vi "_시리얼_Mark10-제어 (압력설정).vi"(3 "FTS 제어 상태":T1="압력제어 시작", 4 "압력 설정(lb)":dbl=10.0 min=0.0 max=160.0 step=0.01 format="%.2f", 5 "시리얼 포트":refnum<visa-resource-name>="COM5") -> (0 "게이지 압력(lb)":dbl min=0.0 max=160.0 step=0.01 format="%.2f", 1 "통신 정상":bool=TRUE, 2 "시리얼 포트out":refnum<visa-resource-name>="COM5")   [LabVIEW 2015]
panel:
  out "미세조정 횟수":u32
  in  "속도-미세조정(mm/min)":dbl=1.0
  in  "속도-저속(mm/min)":dbl=4.0
  in  "속도-중속(mm/min)":dbl=60.0
  in  "속도-고속(mm/min)":dbl=250.0
  # "MARK10 압력 제어"
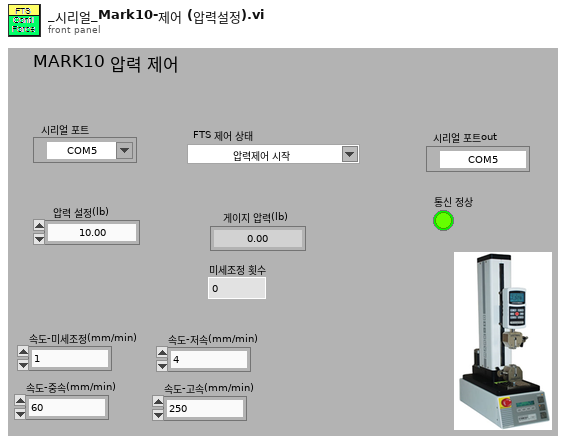
[diagram p1: front panel]
types:
  T1 = typedef "컨트롤-동작상태 FTS.ctl" = string
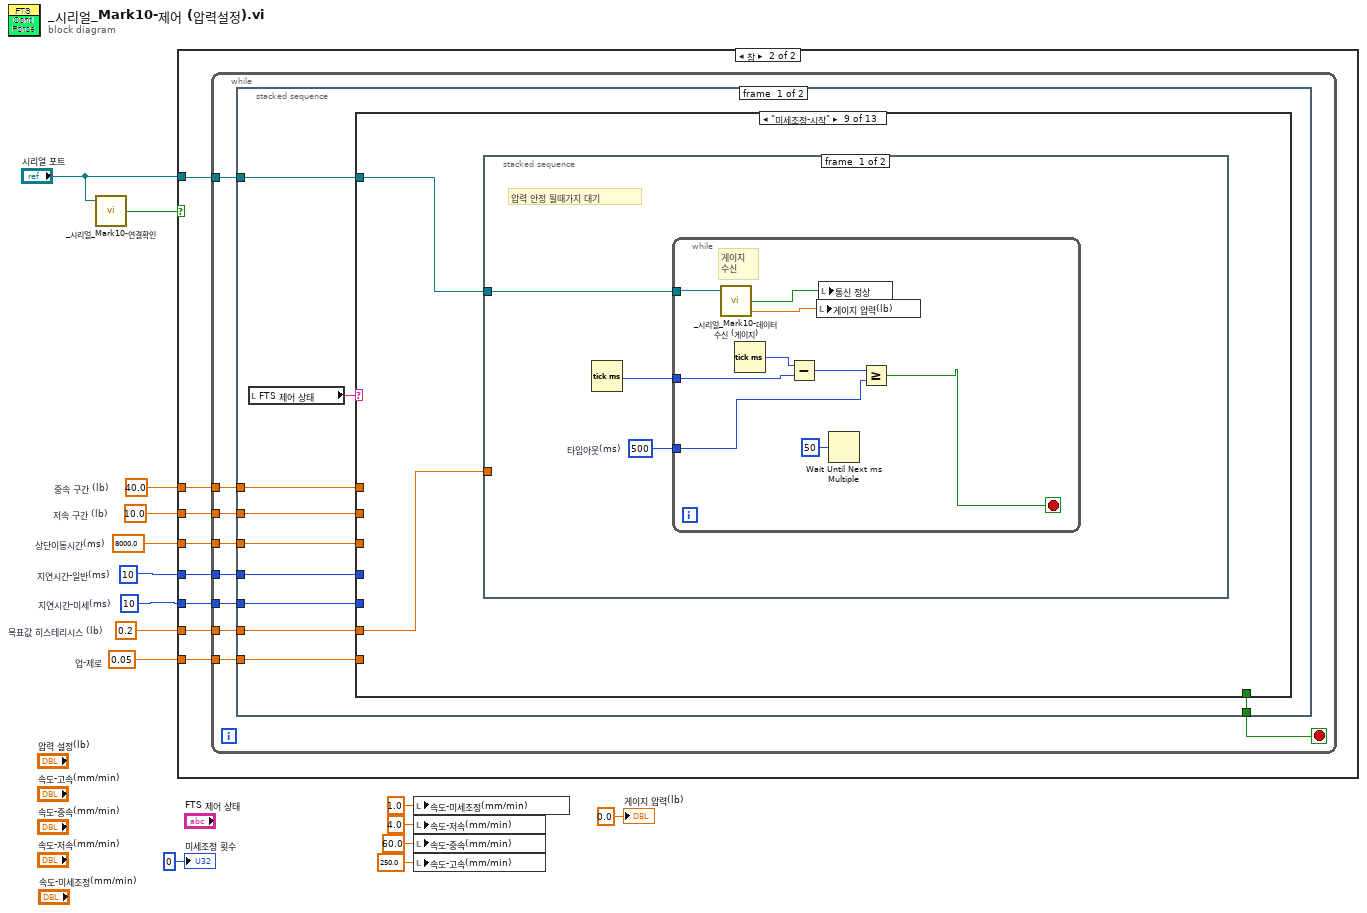
[diagram p0: block diagram]
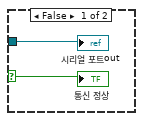
[diagram p2: hidden frame]
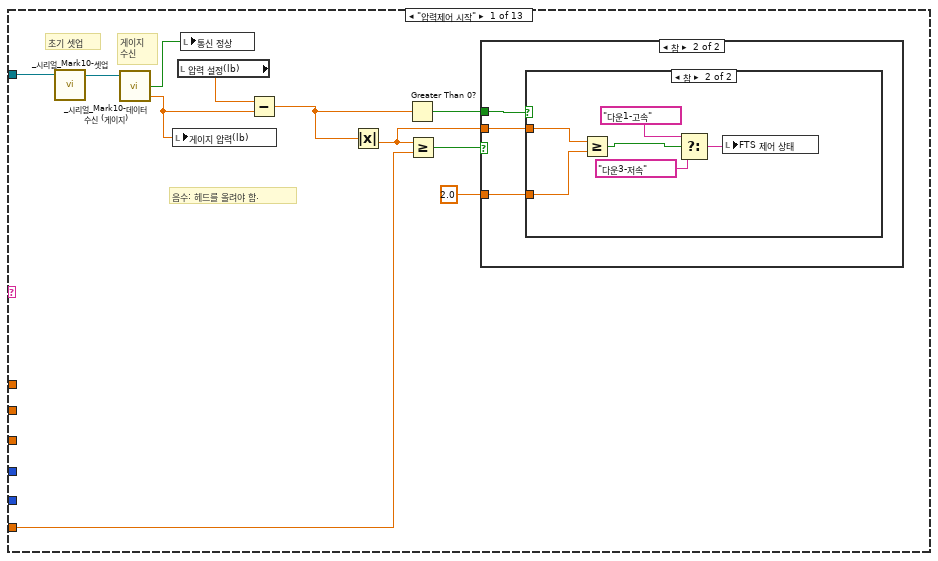
[diagram p3: hidden frame]
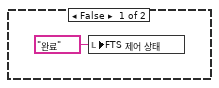
[diagram p4: hidden frame]
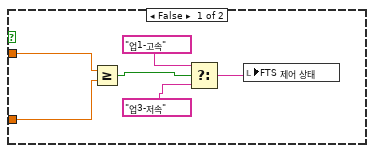
[diagram p5: hidden frame]
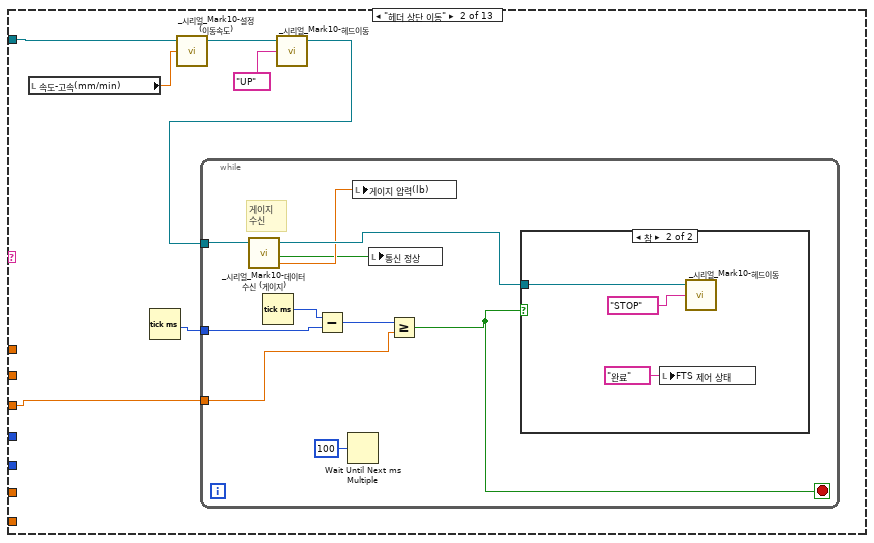
[diagram p6: hidden frame]
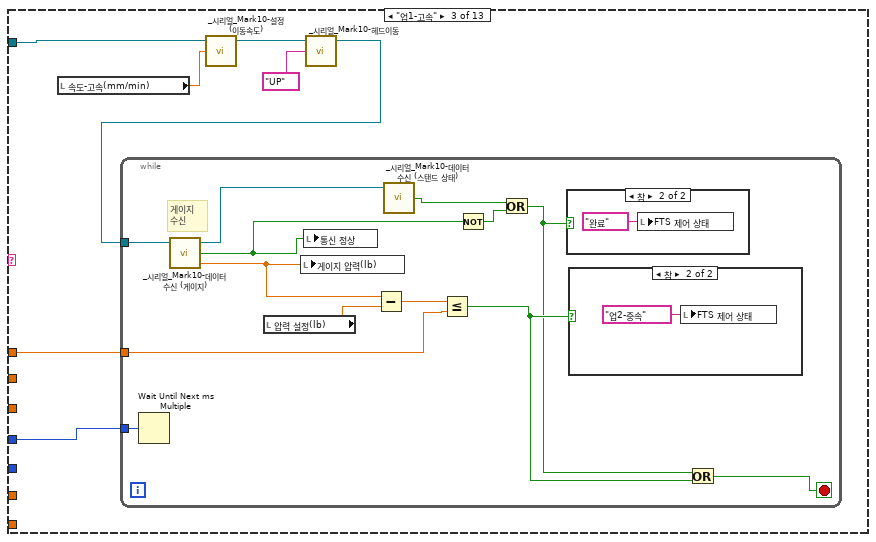
[diagram p8: hidden frame]
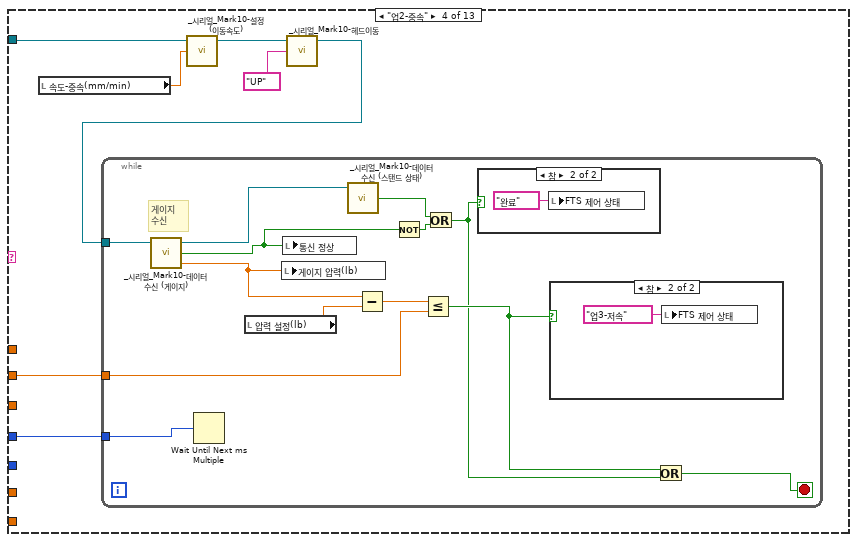
[diagram p11: hidden frame]
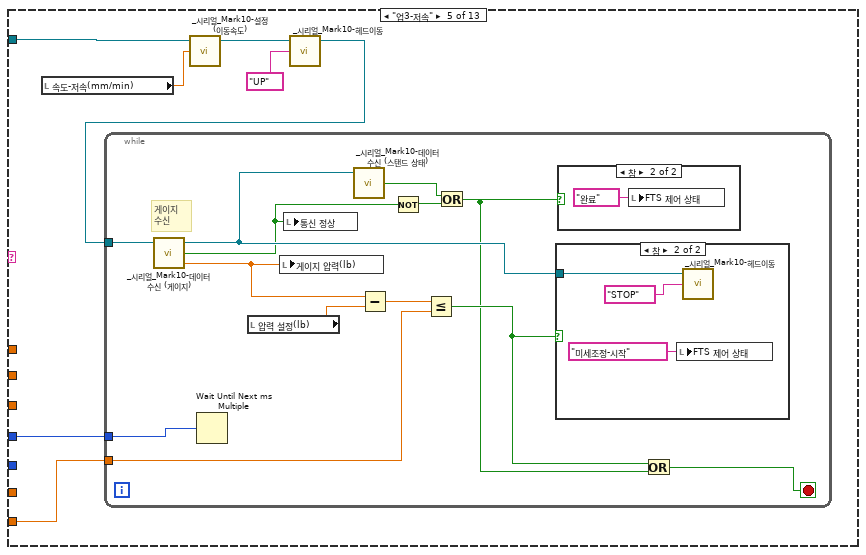
[diagram p14: hidden frame]
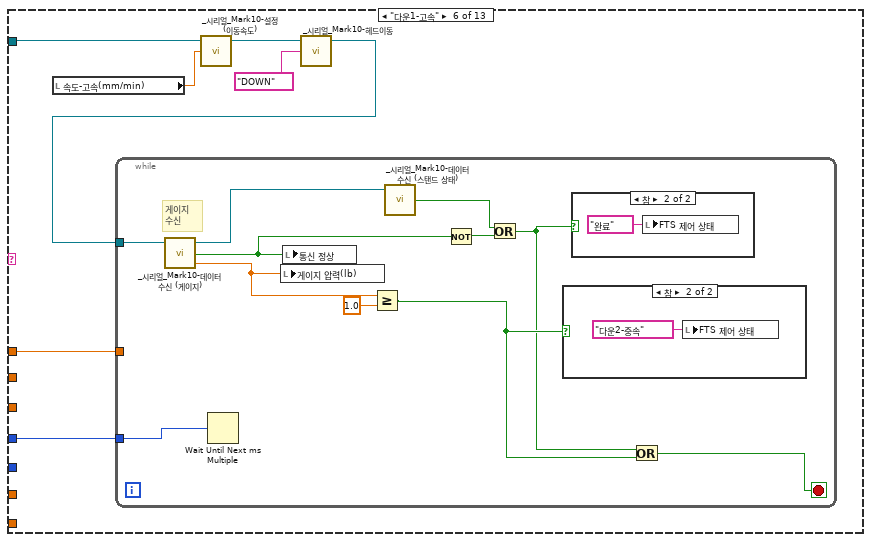
[diagram p17: hidden frame]
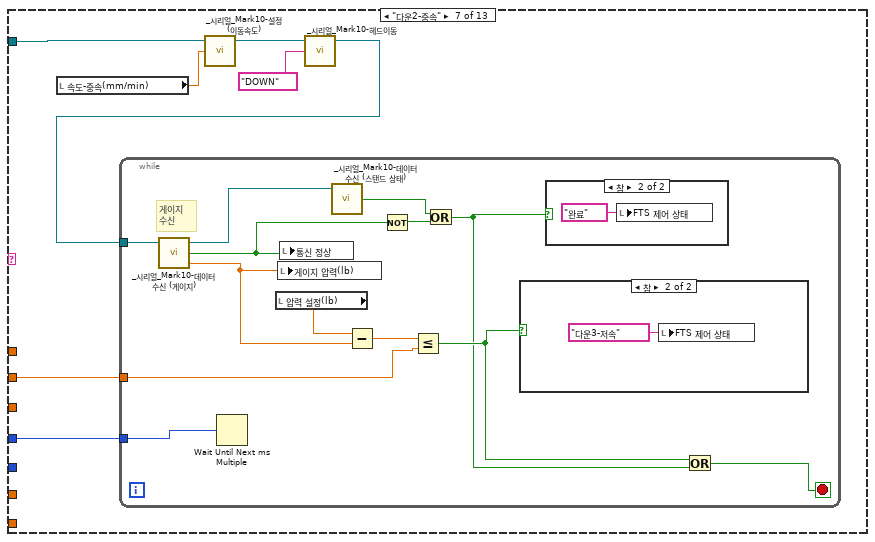
[diagram p20: hidden frame]
diagram:
  w1 = 0.05  # 업-제로
  w3 = 0.2  # 목표값 히스테리시스 (lb)
  w8 = u32 10  # 지연시간-미세(ms)
  w9 = u32 10  # 지연시간-일반(ms)
  w10 = 8000.0  # 상단이동시간(ms)
  w11 = 10.0  # 저속 구간 (lb)
  w12 = 40.0  # 중속 구간 (lb)
  n1 = call "_시리얼_Mark10-연결확인.vi"("시리얼 포트"="시리얼 포트") -> ("수신 정상"=w13:bool)  [unwired: 3 in, 1 out]
  n2 = case shown="참" w13 {
    selector: w13 -> [w16 _]
    tunnel: "시리얼 포트" -> [w17 w25]
    tunnel: w12 -> [_ w24]
    tunnel: w11 -> [_ w23]
    tunnel: w10 -> [_ w22]
    tunnel: w9 -> [_ w21]
    tunnel: w8 -> [_ w20]
    tunnel: w3 -> [_ w19]
    tunnel: w1 -> [_ w18]
    frame False {
      "통신 정상" <- w16
      "시리얼 포트out" <- w17
    }
    frame True {
      n3 = while {
        tunnel: w25 -> [w34]
        tunnel: w24 -> [w32]
        tunnel: w23 -> [w31]
        tunnel: w22 -> [w30]
        tunnel: w21 -> [w29]
        tunnel: w20 -> [w28]
        tunnel: w19 -> [w27]
        tunnel: w18 -> [w26]
        stop <- w33 stop-if-true
        n4 = stacked-sequence {
          tunnel: w34 -> [w44 _]
          tunnel: [w42 _] -> w33
          tunnel: w32 -> [w41 _]
          tunnel: w31 -> [w40 _]
          tunnel: w30 -> [w39 _]
          tunnel: w29 -> [w38 _]
          tunnel: w28 -> [w37 _]
          tunnel: w27 -> [w36 _]
          tunnel: w26 -> [w35 _]
          frame #0 {
            n5 = local read "FTS 제어 상태"() -> (w43:T1)
            n6 = case shown="\"미세조정-시작\"" w43 {
              tunnel: w44 -> [w55 w74 w94 w116 w138 w165 w182 w203 w226 w254 w279 w304 w325]
              tunnel: [_ _ _ _ _ _ _ _ _ _ _ _ TRUE] -> w42
              tunnel: w41 -> [_ _ w93 _ _ w161 _ _ _ _ _ _ _]
              tunnel: w40 -> [_ _ _ w115 _ _ w181 _ _ _ _ _ _]
              tunnel: w39 -> [_ w72 _ _ _ _ _ _ _ _ _ _ _]
              tunnel: w38 -> [_ _ w92 w114 w137 w160 w180 w202 _ _ _ _ _]
              tunnel: w37 -> [_ _ _ _ _ _ _ _ _ w253 w278 _ _]
              tunnel: w36 -> [w45 _ _ _ _ _ _ _ w225 _ _ w303 _]
              tunnel: w35 -> [_ _ _ _ w136 _ _ _ _ _ w277 _ _]
              frame "압력제어 시작" {
                # "음수: 헤드를 올려야 함."
                # "게이지\n수신"
                # "초기 셋업"
                n7 = call "_시리얼_Mark10-셋업.vi"("시리얼 포트"=w55) -> ("VISA 리소스 이름 출력"=w54:refnum<visa-resource-name>)  [unwired: 4 in]
                n8 = call "_시리얼_Mark10-데이터 수신 (게이지).vi"("시리얼 포트"=w54) -> ("데이터(lb)"=w52:dbl, "수신 정상"=w46:bool)  [unwired: 2 in, 1 out]
                n9 = local write "게이지 압력(lb)"(w52) -> ()
                n10 = local read "압력 설정(lb)"() -> (w53:dbl)
                n11 = local write "통신 정상"(w46) -> ()
                n12 = Subtract(x=w53, y=w52) -> (x-y=w50:dbl)
                n13 = Absolute Value(x=w50) -> (abs(x)=w48:dbl)
                n14 = Greater Than 0?(x=w50) -> (x > 0?=w49:bool)
                n15 = Greater Or Equal?(x=w48, y=w45) -> (x >= y?=w51:bool)
                n16 = case shown="참" w51 {
                  tunnel: w49 -> [_ w59]
                  tunnel: w48 -> [_ w58]
                  tunnel: 2.0 ("y") -> [_ w57]
                  frame False {
                    n17 = local write "FTS 제어 상태"(T1 "완료" ("FTS 제어 상태")) -> ()
                  }
                  frame True {
                    n18 = case shown="참" w59 {
                      tunnel: w58 -> [w62 w71]
                      tunnel: w57 -> [w60 w67]
                      frame False {
                        n19 = Greater Or Equal?(x=w62, y=w60) -> (x >= y?=w65:bool)
                        n20 = Select(t=T1 "업1-고속" ("FTS 제어 상태"), s=w65, f=T1 "업3-저속" ("FTS 제어 상태")) -> (s? t:f=w61:T1)
                        n21 = local write "FTS 제어 상태"(w61) -> ()
                      }
                      frame True {
                        n22 = Greater Or Equal?(x=w71, y=w67) -> (x >= y?=w70:bool)
                        n23 = Select(t=T1 "다운1-고속" ("FTS 제어 상태"), s=w70, f=T1 "다운3-저속") -> (s? t:f=w68:T1)
                        n24 = local write "FTS 제어 상태"(w68) -> ()
                      }
                    }
                  }
                }
              }
              frame "헤더 상단 이동" {
                n25 = local read "속도-고속(mm/min)"() -> (w78:dbl)
                n26 = Tick Count (ms)() -> (millisecond timer value=w73:u32)
                n27 = call "_시리얼_Mark10-설정 (이동속도).vi"("속도(mm/min)"=w78, "시리얼 포트"=w74) -> ("VISA 리소스 이름 출력"=w76:refnum<visa-resource-name>)  [unwired: 3 in]
                n28 = call "_시리얼_Mark10-헤드이동.vi"("동작 모드"="UP", "시리얼 포트"=w76) -> ("VISA 리소스 이름 출력"=w75:refnum<visa-resource-name>)  [unwired: 3 in]
                n29 = while {
                  tunnel: w75 -> [w88]
                  tunnel: w73 -> [w83]
                  tunnel: w72 -> [w81]
                  stop <- w80 stop-if-true
                  # "게이지\n수신"
                  n30 = call "_시리얼_Mark10-데이터 수신 (게이지).vi"("시리얼 포트"=w88) -> ("데이터(lb)"=w85:dbl, "수신 정상"=w79:bool, "시리얼 포트 out"=w87:refnum<visa-resource-name>)  [unwired: 2 in]
                  n31 = Tick Count (ms)() -> (millisecond timer value=w84:u32)
                  n32 = Subtract(x=w84, y=w83) -> (x-y=w82:u32)
                  n33 = Wait Until Next ms Multiple(millisecond multiple=u32 100 ("ms 배수")) -> ()  [unwired: 1 out]
                  n34 = local write "게이지 압력(lb)"(w85) -> ()
                  n35 = local write "통신 정상"(w79) -> ()
                  n36 = Greater Or Equal?(x=w82, y=w81) -> (x >= y?=w80:bool)
                  n37 = case shown="참" w80 {
                    tunnel: w87 -> [_ w89]
                    frame False {
                    }
                    frame True {
                      n38 = local write "FTS 제어 상태"(T1 "완료" ("FTS 제어 상태")) -> ()
                      n39 = call "_시리얼_Mark10-헤드이동.vi"("동작 모드"="STOP", "시리얼 포트"=w89) -> ()  [unwired: 3 in, 1 out]
                    }
                  }
                }
              }
              frame "업1-고속" {
                n40 = local read "속도-고속(mm/min)"() -> (w98:dbl)
                n41 = call "_시리얼_Mark10-설정 (이동속도).vi"("속도(mm/min)"=w98, "시리얼 포트"=w94) -> ("VISA 리소스 이름 출력"=w96:refnum<visa-resource-name>)  [unwired: 3 in]
                n42 = call "_시리얼_Mark10-헤드이동.vi"("동작 모드"="UP", "시리얼 포트"=w96) -> ("VISA 리소스 이름 출력"=w95:refnum<visa-resource-name>)  [unwired: 3 in]
                n43 = while {
                  tunnel: w95 -> [w111]
                  tunnel: w93 -> [w107]
                  tunnel: w92 -> [w106]
                  stop <- w103 stop-if-true
                  # "게이지\n수신"
                  n44 = Wait Until Next ms Multiple(millisecond multiple=w106) -> ()  [unwired: 1 out]
                  n45 = call "_시리얼_Mark10-데이터 수신 (게이지).vi"("시리얼 포트"=w111) -> ("데이터(lb)"=w108:dbl, "수신 정상"=w99:bool, "시리얼 포트 out"=w105:refnum<visa-resource-name>)  [unwired: 2 in]
                  n46 = local read "압력 설정(lb)"() -> (w110:dbl)
                  n47 = local write "게이지 압력(lb)"(w108) -> ()
                  n48 = local write "통신 정상"(w99) -> ()
                  n49 = Subtract(x=w108, y=w110) -> (x-y=w109:dbl)
                  n50 = call "_시리얼_Mark10-데이터 수신 (스탠드 상태).vi"("시리얼 포트"=w105) -> ("모터 정지 상태"=w101:bool)  [unwired: 3 in, 1 out]
                  n51 = Less Or Equal?(x=w109, y=w107) -> (x <= y?=w104:bool)
                  n52 = Not(x=w99) -> (.not. x?=w100:bool)
                  n53 = Or(x=w101, y=w100) -> (x .or. y?=w102:bool)
                  n54 = case shown="참" w102 {
                    frame False {
                    }
                    frame True {
                      n55 = local write "FTS 제어 상태"(T1 "완료" ("FTS 제어 상태")) -> ()
                    }
                  }
                  n56 = case shown="참" w104 {
                    frame False {
                    }
                    frame True {
                      n57 = local write "FTS 제어 상태"(T1 "업2-중속" ("FTS 제어 상태")) -> ()
                    }
                  }
                  n58 = Or(x=w102, y=w104) -> (x .or. y?=w103:bool)
                }
              }
              frame "업2-중속" {
                n59 = local read "속도-중속(mm/min)"() -> (w120:dbl)
                n60 = call "_시리얼_Mark10-설정 (이동속도).vi"("속도(mm/min)"=w120, "시리얼 포트"=w116) -> ("VISA 리소스 이름 출력"=w118:refnum<visa-resource-name>)  [unwired: 3 in]
                n61 = call "_시리얼_Mark10-헤드이동.vi"("동작 모드"="UP", "시리얼 포트"=w118) -> ("VISA 리소스 이름 출력"=w117:refnum<visa-resource-name>)  [unwired: 3 in]
                n62 = while {
                  tunnel: w117 -> [w133]
                  tunnel: w115 -> [w129]
                  tunnel: w114 -> [w128]
                  stop <- w125 stop-if-true
                  # "게이지\n수신"
                  n63 = call "_시리얼_Mark10-데이터 수신 (게이지).vi"("시리얼 포트"=w133) -> ("데이터(lb)"=w130:dbl, "수신 정상"=w121:bool, "시리얼 포트 out"=w127:refnum<visa-resource-name>)  [unwired: 2 in]
                  n64 = Wait Until Next ms Multiple(millisecond multiple=w128) -> ()  [unwired: 1 out]
                  n65 = local read "압력 설정(lb)"() -> (w132:dbl)
                  n66 = local write "게이지 압력(lb)"(w130) -> ()
                  n67 = local write "통신 정상"(w121) -> ()
                  n68 = call "_시리얼_Mark10-데이터 수신 (스탠드 상태).vi"("시리얼 포트"=w127) -> ("모터 정지 상태"=w123:bool)  [unwired: 3 in, 1 out]
                  n69 = Subtract(x=w130, y=w132) -> (x-y=w131:dbl)
                  n70 = Not(x=w121) -> (.not. x?=w124:bool)
                  n71 = Less Or Equal?(x=w131, y=w129) -> (x <= y?=w126:bool)
                  n72 = Or(x=w123, y=w124) -> (x .or. y?=w122:bool)
                  n73 = case shown="참" w122 {
                    frame False {
                    }
                    frame True {
                      n74 = local write "FTS 제어 상태"(T1 "완료" ("FTS 제어 상태")) -> ()
                    }
                  }
                  n75 = case shown="참" w126 {
                    frame False {
                    }
                    frame True {
                      n76 = local write "FTS 제어 상태"(T1 "업3-저속" ("FTS 제어 상태")) -> ()
                    }
                  }
                  n77 = Or(x=w126, y=w122) -> (x .or. y?=w125:bool)
                }
              }
              frame "업3-저속" {
                n78 = local read "속도-저속(mm/min)"() -> (w142:dbl)
                n79 = call "_시리얼_Mark10-설정 (이동속도).vi"("속도(mm/min)"=w142, "시리얼 포트"=w138) -> ("VISA 리소스 이름 출력"=w140:refnum<visa-resource-name>)  [unwired: 3 in]
                n80 = call "_시리얼_Mark10-헤드이동.vi"("동작 모드"="UP", "시리얼 포트"=w140) -> ("VISA 리소스 이름 출력"=w139:refnum<visa-resource-name>)  [unwired: 3 in]
                n81 = while {
                  tunnel: w139 -> [w155]
                  tunnel: w137 -> [w151]
                  tunnel: w136 -> [w143]
                  stop <- w148 stop-if-true
                  # "게이지\n수신"
                  n82 = call "_시리얼_Mark10-데이터 수신 (게이지).vi"("시리얼 포트"=w155) -> ("데이터(lb)"=w152:dbl, "수신 정상"=w147:bool, "시리얼 포트 out"=w150:refnum<visa-resource-name>)  [unwired: 2 in]
                  n83 = Wait Until Next ms Multiple(millisecond multiple=w151) -> ()  [unwired: 1 out]
                  n84 = local read "압력 설정(lb)"() -> (w154:dbl)
                  n85 = local write "게이지 압력(lb)"(w152) -> ()
                  n86 = local write "통신 정상"(w147) -> ()
                  n87 = call "_시리얼_Mark10-데이터 수신 (스탠드 상태).vi"("시리얼 포트"=w150) -> ("모터 정지 상태"=w145:bool)  [unwired: 3 in, 1 out]
                  n88 = Subtract(x=w152, y=w154) -> (x-y=w153:dbl)
                  n89 = Not(x=w147) -> (.not. x?=w146:bool)
                  n90 = Less Or Equal?(x=w153, y=w143) -> (x <= y?=w149:bool)
                  n91 = Or(x=w145, y=w146) -> (x .or. y?=w144:bool)
                  n92 = case shown="참" w149 {
                    tunnel: w150 -> [_ w158]
                    frame False {
                    }
                    frame True {
                      n93 = local write "FTS 제어 상태"(T1 "미세조정-시작" ("FTS 제어 상태")) -> ()
                      n94 = call "_시리얼_Mark10-헤드이동.vi"("동작 모드"="STOP", "시리얼 포트"=w158) -> ()  [unwired: 3 in, 1 out]
                    }
                  }
                  n95 = case shown="참" w144 {
                    frame False {
                    }
                    frame True {
                      n96 = local write "FTS 제어 상태"(T1 "완료" ("FTS 제어 상태")) -> ()
                    }
                  }
                  n97 = Or(x=w149, y=w144) -> (x .or. y?=w148:bool)
                }
              }
              frame "다운1-고속" {
                n98 = local read "속도-고속(mm/min)"() -> (w166:dbl)
                n99 = call "_시리얼_Mark10-설정 (이동속도).vi"("속도(mm/min)"=w166, "시리얼 포트"=w165) -> ("VISA 리소스 이름 출력"=w163:refnum<visa-resource-name>)  [unwired: 3 in]
                n100 = call "_시리얼_Mark10-헤드이동.vi"("동작 모드"="DOWN", "시리얼 포트"=w163) -> ("VISA 리소스 이름 출력"=w162:refnum<visa-resource-name>)  [unwired: 3 in]
                n101 = while {
                  tunnel: w162 -> [w177]
                  tunnel: w161 -> [_]
                  tunnel: w160 -> [w174]
                  stop <- w171 stop-if-true
                  # "게이지\n수신"
                  n102 = call "_시리얼_Mark10-데이터 수신 (게이지).vi"("시리얼 포트"=w177) -> ("데이터(lb)"=w176:dbl, "수신 정상"=w170:bool, "시리얼 포트 out"=w173:refnum<visa-resource-name>)  [unwired: 2 in]
                  n103 = Wait Until Next ms Multiple(millisecond multiple=w174) -> ()  [unwired: 1 out]
                  n104 = local write "게이지 압력(lb)"(w176) -> ()
                  n105 = local write "통신 정상"(w170) -> ()
                  n106 = Greater Or Equal?(x=w176, y=1.0) -> (x >= y?=w172:bool)
                  n107 = call "_시리얼_Mark10-데이터 수신 (스탠드 상태).vi"("시리얼 포트"=w173) -> ("모터 정지 상태"=w168:bool)  [unwired: 3 in, 1 out]
                  n108 = Not(x=w170) -> (.not. x?=w169:bool)
                  n109 = Or(x=w168, y=w169) -> (x .or. y?=w167:bool)
                  n110 = case shown="참" w172 {
                    frame False {
                    }
                    frame True {
                      n111 = local write "FTS 제어 상태"(T1 "다운2-중속" ("FTS 제어 상태")) -> ()
                    }
                  }
                  n112 = case shown="참" w167 {
                    frame False {
                    }
                    frame True {
                      n113 = local write "FTS 제어 상태"(T1 "완료" ("FTS 제어 상태")) -> ()
                    }
                  }
                  n114 = Or(x=w167, y=w172) -> (x .or. y?=w171:bool)
                }
              }
              frame "다운2-중속" {
                n115 = local read "속도-중속(mm/min)"() -> (w186:dbl)
                n116 = call "_시리얼_Mark10-설정 (이동속도).vi"("속도(mm/min)"=w186, "시리얼 포트"=w182) -> ("VISA 리소스 이름 출력"=w184:refnum<visa-resource-name>)  [unwired: 3 in]
                n117 = call "_시리얼_Mark10-헤드이동.vi"("동작 모드"="DOWN", "시리얼 포트"=w184) -> ("VISA 리소스 이름 출력"=w183:refnum<visa-resource-name>)  [unwired: 3 in]
                n118 = while {
                  tunnel: w183 -> [w199]
                  tunnel: w181 -> [w195]
                  tunnel: w180 -> [w194]
                  stop <- w191 stop-if-true
                  # "게이지\n수신"
                  n119 = call "_시리얼_Mark10-데이터 수신 (게이지).vi"("시리얼 포트"=w199) -> ("데이터(lb)"=w196:dbl, "수신 정상"=w190:bool, "시리얼 포트 out"=w193:refnum<visa-resource-name>)  [unwired: 2 in]
                  n120 = Wait Until Next ms Multiple(millisecond multiple=w194) -> ()  [unwired: 1 out]
                  n121 = local read "압력 설정(lb)"() -> (w198:dbl)
                  n122 = local write "게이지 압력(lb)"(w196) -> ()
                  n123 = local write "통신 정상"(w190) -> ()
                  n124 = call "_시리얼_Mark10-데이터 수신 (스탠드 상태).vi"("시리얼 포트"=w193) -> ("모터 정지 상태"=w188:bool)  [unwired: 3 in, 1 out]
                  n125 = Subtract(x=w198, y=w196) -> (x-y=w197:dbl)
                  n126 = Not(x=w190) -> (.not. x?=w189:bool)
                  n127 = Less Or Equal?(x=w197, y=w195) -> (x <= y?=w192:bool)
                  n128 = Or(x=w188, y=w189) -> (x .or. y?=w187:bool)
                  n129 = case shown="참" w192 {
                    frame False {
                    }
                    frame True {
                      n130 = local write "FTS 제어 상태"(T1 "다운3-저속" ("FTS 제어 상태")) -> ()
                    }
                  }
                  n131 = case shown="참" w187 {
                    frame False {
                    }
                    frame True {
                      n132 = local write "FTS 제어 상태"(T1 "완료" ("FTS 제어 상태")) -> ()
                    }
                  }
                  n133 = Or(x=w192, y=w187) -> (x .or. y?=w191:bool)
                }
              }
              frame "다운3-저속" {
                n134 = local read "속도-저속(mm/min)"() -> (w207:dbl)
                n135 = call "_시리얼_Mark10-설정 (이동속도).vi"("속도(mm/min)"=w207, "시리얼 포트"=w203) -> ("VISA 리소스 이름 출력"=w205:refnum<visa-resource-name>)  [unwired: 3 in]
                n136 = call "_시리얼_Mark10-헤드이동.vi"("동작 모드"="DOWN", "시리얼 포트"=w205) -> ("VISA 리소스 이름 출력"=w204:refnum<visa-resource-name>)  [unwired: 3 in]
                n137 = while {
                  tunnel: w204 -> [w220]
                  tunnel: w202 -> [w216]
                  stop <- w214 stop-if-true
                  # "게이지\n수신"
                  n138 = call "_시리얼_Mark10-데이터 수신 (게이지).vi"("시리얼 포트"=w220) -> ("데이터(lb)"=w217:dbl, "수신 정상"=w208:bool, "시리얼 포트 out"=w213:refnum<visa-resource-name>)  [unwired: 2 in]
                  n139 = Wait Until Next ms Multiple(millisecond multiple=w216) -> ()  [unwired: 1 out]
                  n140 = local write "통신 정상"(w208) -> ()
                  n141 = local read "압력 설정(lb)"() -> (w219:dbl)
                  n142 = local write "게이지 압력(lb)"(w217) -> ()
                  n143 = Subtract(x=w219, y=w217) -> (x-y=w218:dbl)
                  n144 = call "_시리얼_Mark10-데이터 수신 (스탠드 상태).vi"("시리얼 포트"=w213) -> ("모터 정지 상태"=w211:bool, "시리얼 포트 out"=w212:refnum<visa-resource-name>)  [unwired: 3 in]
                  n145 = Less Or Equal To 0?(x=w218) -> (x <= 0?=w215:bool)
                  n146 = Not(x=w208) -> (.not. x?=w210:bool)
                  n147 = Or(x=w211, y=w210) -> (x .or. y?=w209:bool)
                  n148 = case shown="참" w215 {
                    tunnel: w212 -> [_ w223]
                    frame False {
                    }
                    frame True {
                      n149 = local write "FTS 제어 상태"(T1 "미세조정-시작" ("FTS 제어 상태")) -> ()
                      n150 = call "_시리얼_Mark10-헤드이동.vi"("동작 모드"="STOP", "시리얼 포트"=w223) -> ()  [unwired: 3 in, 1 out]
                    }
                  }
                  n151 = case shown="참" w209 {
                    frame False {
                    }
                    frame True {
                      n152 = local write "FTS 제어 상태"(T1 "완료" ("FTS 제어 상태")) -> ()
                    }
                  }
                  n153 = Or(x=w215, y=w209) -> (x .or. y?=w214:bool)
                }
              }
              frame "미세조정-시작" {
                n154 = stacked-sequence {
                  tunnel: w226 -> [w229 w247]
                  tunnel: w225 -> [_ w244]
                  frame #0 {
                    w227 = u32 500  # 타임아웃(ms)
                    # "압력 안정 될때가지 대기"
                    n155 = Tick Count (ms)() -> (millisecond timer value=w228:u32)
                    n156 = while {
                      tunnel: w229 -> [w238]
                      tunnel: w228 -> [w234]
                      tunnel: w227 -> [w232]
                      stop <- w231 stop-if-true
                      # "게이지\n수신"
                      n157 = call "_시리얼_Mark10-데이터 수신 (게이지).vi"("시리얼 포트"=w238) -> ("데이터(lb)"=w236:dbl, "수신 정상"=w230:bool)  [unwired: 2 in, 1 out]
                      n158 = Tick Count (ms)() -> (millisecond timer value=w235:u32)
                      n159 = Subtract(x=w235, y=w234) -> (x-y=w233:u32)
                      n160 = local write "게이지 압력(lb)"(w236) -> ()
                      n161 = local write "통신 정상"(w230) -> ()
                      n162 = Wait Until Next ms Multiple(millisecond multiple=u32 50 ("ms 배수")) -> ()  [unwired: 1 out]
                      n163 = Greater Or Equal?(x=w233, y=w232) -> (x >= y?=w231:bool)
                    }
                  }
                  frame #1 {
                    # "음수: 헤드를 올려야 함."
                    # "게이지\n수신"
                    n164 = call "_시리얼_Mark10-데이터 수신 (게이지).vi"("시리얼 포트"=w247) -> ("데이터(lb)"=w248:dbl, "수신 정상"=w246:bool)  [unwired: 2 in, 1 out]
                    n165 = local write "게이지 압력(lb)"(w248) -> ()
                    n166 = local read "압력 설정(lb)"() -> (w249:dbl)
                    n167 = local write "통신 정상"(w246) -> ()
                    n168 = Subtract(x=w249, y=w248) -> (x-y=w245:dbl)
                    n169 = Multiply(x=w244, y=-1.0) -> (x*y=w243:dbl)
                    n170 = Greater Or Equal?(x=w245, y=w244) -> (x >= y?=w240:bool)
                    n171 = Less Or Equal?(x=w245, y=w243) -> (x <= y?=w241:bool)
                    n172 = Or(x=w241, y=w240) -> (x .or. y?=w239:bool)
                    n173 = case shown="참" w240 {
                      frame False {
                      }
                      frame True {
                        n174 = local write "FTS 제어 상태"(T1 "미세조정-다운" ("FTS 제어 상태")) -> ()
                      }
                    }
                    n175 = case shown="참" w241 {
                      frame False {
                      }
                      frame True {
                        n176 = local write "FTS 제어 상태"(T1 "미세조정-업" ("FTS 제어 상태")) -> ()
                      }
                    }
                    n177 = case shown="거짓" w239 {
                      frame False {
                        n178 = local write "FTS 제어 상태"(T1 "미세조정-종료" ("FTS 제어 상태")) -> ()
                      }
                      frame True {
                      }
                    }
                  }
                }
              }
              frame "미세조정-다운" {
                n179 = local read "속도-미세조정(mm/min)"() -> (w258:dbl)
                n180 = call "_시리얼_Mark10-설정 (이동속도).vi"("속도(mm/min)"=w258, "시리얼 포트"=w254) -> ("VISA 리소스 이름 출력"=w256:refnum<visa-resource-name>)  [unwired: 3 in]
                n181 = call "_시리얼_Mark10-헤드이동.vi"("동작 모드"="DOWN", "시리얼 포트"=w256) -> ("VISA 리소스 이름 출력"=w255:refnum<visa-resource-name>)  [unwired: 3 in]
                n182 = while {
                  tunnel: w255 -> [w271]
                  tunnel: w253 -> [w265]
                  stop <- w266 stop-if-true
                  # "게이지\n수신"
                  n183 = call "_시리얼_Mark10-데이터 수신 (게이지).vi"("시리얼 포트"=w271) -> ("데이터(lb)"=w268:dbl, "수신 정상"=w259:bool, "시리얼 포트 out"=w264:refnum<visa-resource-name>)  [unwired: 2 in]
                  n184 = local write "통신 정상"(w259) -> ()
                  n185 = local read "압력 설정(lb)"() -> (w270:dbl)
                  n186 = local write "게이지 압력(lb)"(w268) -> ()
                  n187 = call "_시리얼_Mark10-데이터 수신 (스탠드 상태).vi"("시리얼 포트"=w264) -> ("모터 정지 상태"=w261:bool, "시리얼 포트 out"=w263:refnum<visa-resource-name>)  [unwired: 3 in]
                  n188 = Subtract(x=w270, y=w268) -> (x-y=w269:dbl)
                  n189 = Not(x=w259) -> (.not. x?=w262:bool)
                  n190 = Less Or Equal To 0?(x=w269) -> (x <= 0?=w267:bool)
                  n191 = Or(x=w261, y=w262) -> (x .or. y?=w260:bool)
                  n192 = case shown="참" w267 {
                    tunnel: w263 -> [_ w275]
                    tunnel: w265 -> [w273 _]
                    frame False {
                      n193 = Wait Until Next ms Multiple(millisecond multiple=w273) -> ()  [unwired: 1 out]
                    }
                    frame True {
                      n194 = local write "FTS 제어 상태"(T1 "미세조정-종료" ("FTS 제어 상태")) -> ()
                      n195 = call "_시리얼_Mark10-헤드이동.vi"("동작 모드"="STOP", "시리얼 포트"=w275) -> ()  [unwired: 3 in, 1 out]
                    }
                  }
                  n196 = case shown="참" w260 {
                    frame False {
                    }
                    frame True {
                      n197 = local write "FTS 제어 상태"(T1 "완료" ("FTS 제어 상태")) -> ()
                    }
                  }
                  n198 = Or(x=w267, y=w260) -> (x .or. y?=w266:bool)
                }
              }
              frame "미세조정-업" {
                n199 = local read "속도-저속(mm/min)"() -> (w283:dbl)
                n200 = call "_시리얼_Mark10-설정 (이동속도).vi"("속도(mm/min)"=w283, "시리얼 포트"=w279) -> ("VISA 리소스 이름 출력"=w281:refnum<visa-resource-name>)  [unwired: 3 in]
                n201 = call "_시리얼_Mark10-헤드이동.vi"("동작 모드"="UP", "시리얼 포트"=w281) -> ("VISA 리소스 이름 출력"=w280:refnum<visa-resource-name>)  [unwired: 3 in]
                n202 = while {
                  tunnel: w280 -> [w297]
                  tunnel: w278 -> [w291]
                  tunnel: w277 -> [w284]
                  stop <- w292 stop-if-true
                  # "게이지\n수신"
                  n203 = call "_시리얼_Mark10-데이터 수신 (게이지).vi"("시리얼 포트"=w297) -> ("데이터(lb)"=w294:dbl, "수신 정상"=w286:bool, "시리얼 포트 out"=w290:refnum<visa-resource-name>)  [unwired: 2 in]
                  n204 = local read "압력 설정(lb)"() -> (w296:dbl)
                  n205 = local write "게이지 압력(lb)"(w294) -> ()
                  n206 = local write "통신 정상"(w286) -> ()
                  n207 = call "_시리얼_Mark10-데이터 수신 (스탠드 상태).vi"("시리얼 포트"=w290) -> ("모터 정지 상태"=w288:bool, "시리얼 포트 out"=w289:refnum<visa-resource-name>)  [unwired: 3 in]
                  n208 = Subtract(x=w294, y=w296) -> (x-y=w295:dbl)
                  n209 = Not(x=w286) -> (.not. x?=w287:bool)
                  n210 = Less Or Equal?(x=w295, y=w284) -> (x <= y?=w293:bool)
                  n211 = Or(x=w288, y=w287) -> (x .or. y?=w285:bool)
                  n212 = case shown="참" w285 {
                    frame False {
                    }
                    frame True {
                      n213 = local write "FTS 제어 상태"(T1 "완료" ("FTS 제어 상태")) -> ()
                    }
                  }
                  n214 = case shown="참" w293 {
                    tunnel: w289 -> [_ w301]
                    tunnel: w291 -> [w299 _]
                    frame False {
                      n215 = Wait Until Next ms Multiple(millisecond multiple=w299) -> ()  [unwired: 1 out]
                    }
                    frame True {
                      n216 = call "_시리얼_Mark10-헤드이동.vi"("동작 모드"="STOP", "시리얼 포트"=w301) -> ()  [unwired: 3 in, 1 out]
                      n217 = local write "FTS 제어 상태"(T1 "미세조정-종료" ("FTS 제어 상태")) -> ()
                    }
                  }
                  n218 = Or(x=w293, y=w285) -> (x .or. y?=w292:bool)
                }
              }
              frame "미세조정-종료" {
                n219 = stacked-sequence {
                  tunnel: w304 -> [_ w308]
                  tunnel: w303 -> [_ w306]
                  frame #0 {
                    n220 = Wait Until Next ms Multiple(millisecond multiple=u32 1000 ("ms 배수")) -> ()  [unwired: 1 out]
                  }
                  frame #1 {
                    # "게이지\n수신"
                    n221 = call "_시리얼_Mark10-데이터 수신 (게이지).vi"("시리얼 포트"=w308) -> ("데이터(lb)"=w312:dbl, "수신 정상"=w307:bool)  [unwired: 2 in, 1 out]
                    n222 = local write "게이지 압력(lb)"(w312) -> ()
                    n223 = local read "압력 설정(lb)"() -> (w313:dbl)
                    n224 = local write "통신 정상"(w307) -> ()
                    n225 = Subtract(x=w313, y=w312) -> (x-y=w310:dbl)
                    n226 = Absolute Value(x=w310) -> (abs(x)=w309:dbl)
                    n227 = Greater Or Equal?(x=w309, y=w306) -> (x >= y?=w311:bool)
                    n228 = case shown="참" w311 {
                      frame False {
                        # "목표치 도달"
                        n229 = local read "미세조정 횟수"() -> (w317:u32)
                        n230 = Increment(x=w317) -> (x+1=w316:u32)
                        n231 = Greater Or Equal?(x=w316, y=u32 2) -> (x >= y?=w314:bool)
                        n232 = case shown="거짓" w314 {
                          frame False {
                            n233 = local write "FTS 제어 상태"(T1 "미세조정-시작" ("FTS 제어 상태")) -> ()
                          }
                          frame True {
                            n234 = local write "FTS 제어 상태"(T1 "완료" ("FTS 제어 상태")) -> ()
                          }
                        }
                        n235 = local write "미세조정 횟수"(w316) -> ()
                      }
                      frame True {
                        n236 = local write "미세조정 횟수"(u32 0 ("미세조정 횟수")) -> ()
                        n237 = local write "FTS 제어 상태"(T1 "미세조정-시작" ("FTS 제어 상태")) -> ()
                      }
                    }
                  }
                }
              }
              frame "완료", Default {
                n238 = call "_시리얼_Mark10-헤드이동.vi"("동작 모드"="STOP", "시리얼 포트"=w325) -> ("VISA 리소스 이름 출력"=w323:refnum<visa-resource-name>)  [unwired: 3 in]
                n239 = local write "시리얼 포트out"(w323) -> ()
                n240 = local write "FTS 제어 상태"(T1 "압력제어 시작" ("FTS 제어 상태")) -> ()
              }
            }
          }
          frame #1 {
            n241 = local read "통신 정상"() -> (w327:bool)
            n242 = case shown="참" w327 {
              frame False {
                # "통신 에러"
                n243 = local write "FTS 제어 상태"(T1 "완료" ("FTS 제어 상태")) -> ()
              }
              frame True {
              }
            }
          }
        }
      }
    }
  }
  n244 = local write "속도-미세조정(mm/min)"(1.0 ("속도-미세조정(mm/min)")) -> ()
  n245 = local write "속도-저속(mm/min)"(4.0 ("속도-저속(mm/min)")) -> ()
  n246 = local write "속도-중속(mm/min)"(60.0 ("속도-중속(mm/min)")) -> ()
  n247 = local write "속도-고속(mm/min)"(250.0 ("속도-고속(mm/min)")) -> ()
  "게이지 압력(lb)" <- 0.0 ("게이지 압력(lb)")
  "미세조정 횟수" <- u32 0 ("지연시간-미세(ms)")
